vi "Get 1D U64.vi"(5 "format string (%_20f)":string="%_20f", 7 "key description":string, 8 "sections":string[](array[string]), 9 "numeric":u64[](array[numeric]), 11 "info data":string) -> (0 "sections out":string[](array[string]), 2 "value":u64[](array[numeric]), 3 "info data out":string)   [LabVIEW 2013, in "infolib.lvlib"]
doc: "Add a new numeric key to Info Data string. If section exists in Info Data string, inserts key into this section."
uses:
  infolib.lvlib
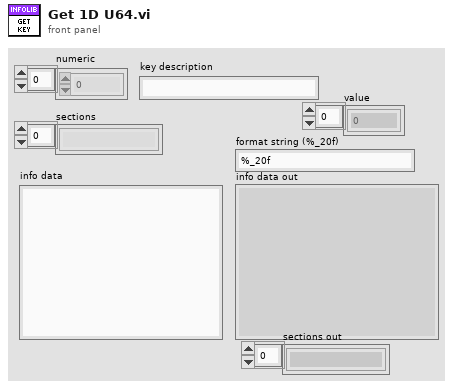
[diagram p1: front panel]
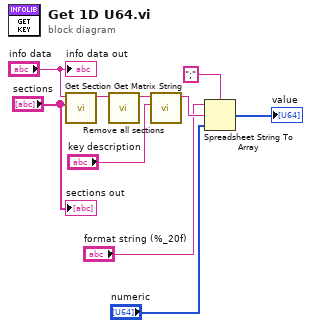
[diagram p0: block diagram]
diagram:
  n1 = call "Get Section.vi"("sections"="sections", "info data"="info data") -> ("section part"=w10:string)  [unwired: 8 in, 1 out]
  n2 = call "Remove all sections.vi"("info data"=w10) -> ("info data out"=w7:string)  [unwired: 10 in]
  n3 = call "Get Matrix String.vi"("matrix key"="key description", "info data"=w7) -> ("matrix part"=w4:string)  [unwired: 8 in, 1 out]
  n4 = Spreadsheet String To Array(delimiter (Tab)=";", format string="format string (%_20f)", spreadsheet string=w4, array type (2D Dbl)="numeric") -> (array=→"value":u64[])
  "info data out" <- "info data"
  "sections out" <- "sections"
